vi "Run Command.vi"(2 "Line Index In":i32, 3 "Script":string) -> (0 "Line Index Out":i32, 1 "Done":bool)   [LabVIEW 2015]
doc: "Looks at a line and runs the appropriate command. Add new commands to this vi."
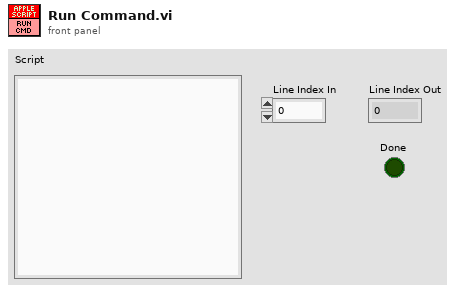
[diagram p1: front panel]
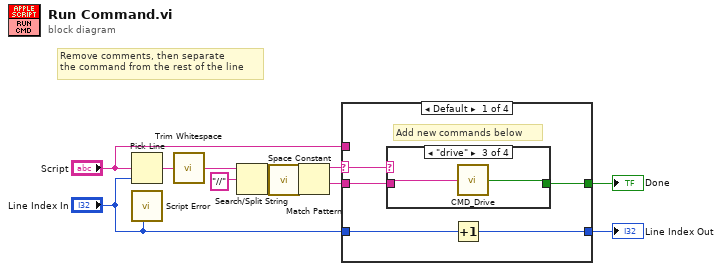
[diagram p0: block diagram]
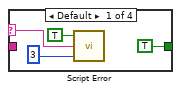
[diagram p2: hidden frame]
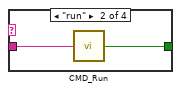
[diagram p3: hidden frame]
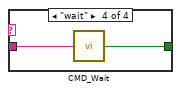
[diagram p4: hidden frame]
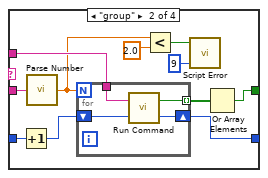
[diagram p5: hidden frame]
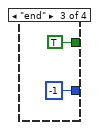
[diagram p6: hidden frame]
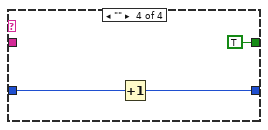
[diagram p7: hidden frame]
diagram:
  # "Remove comments, then separate\nthe command from the rest of the line"
  n1 = Pick Line(multi-line string="Script", line index="Line Index In") -> (output string=w6:string)  [unwired: 1 in]
  n2 = call "Script Error.vi"("Line Number"="Line Index In") -> ()  [unwired: 4 in, 1 out]
  n3 = call <vilib>:"Trim Whitespace.vi"("string"=w6) -> ("trimmed string"=w4:string)  [unwired: 1 in]
  n4 = Search/Split String(string=w4, search string/char (-)="//") -> (substring before match=w3:string)  [unwired: 1 in, 2 out]
  n5 = call <vilib>:"Space Constant.vi"() -> ("String"=w11:string)
  n6 = Match Pattern(string=w3, regular expression=w11) -> (before substring=w2:string, after substring=w1:string)  [unwired: 1 in, 2 out]
  n7 = case shown="Default" w2 {
    selector: w2 -> [w14 _ _ _]
    tunnel: "Script" -> [_ w37 _ _]
    tunnel: "Line Index In" -> [w16 w33 _ w45]
    tunnel: [w13 w35 TRUE ("Running") TRUE ("Running")] -> w9
    tunnel: [w15 w34 -1 ("Line Index Out") w44] -> w8
    tunnel: w1 -> [w12 w27 _ _]
    frame Default {
      # "Add new commands below"
      n8 = case shown="\"drive\"" w14 {
        selector: w14 -> [w17 _ _ _]
        tunnel: [TRUE w21 w23 w26] -> w13
        tunnel: w12 -> [_ w22 w24 w25]
        frame Default {
          n9 = call "Script Error.vi"("Error?"=TRUE, "Error Details"=w17, "Error Code"=3) -> ()  [unwired: 2 in, 1 out]
        }
        frame "run" {
          n10 = call "CMD_Run.vi"("Line"=w22) -> ("Done"=w21:bool)
        }
        frame "drive" {
          n11 = call "CMD_Drive.vi"("Line"=w24) -> ("Done"=w23:bool)
        }
        frame "wait" {
          n12 = call "CMD_Wait.vi"("Line"=w25) -> ("Done"=w26:bool)
        }
      }
      n13 = Increment(x=w16) -> (x+1=w15:i32)
    }
    frame "group" {
      n14 = Increment(x=w33) -> (x+1=w32:i32)
      n15 = call "Parse Number.vi"("String"=w27) -> ("Number"=w30:dbl)
      n16 = for {
        N: w30 -> [_]
        tunnel: w37 -> [w41]
        tunnel: [w40] -> w36 mode=indexing
        shift-right: [w39] -> w34
        shift-left: w32 -> [w38]
        n17 = call "Run Command.vi"("Line Index In"=w38, "Script"=w41) -> ("Line Index Out"=w39:i32, "Done"=w40:bool)
      }
      n18 = Less?(x=w30, y=2.0) -> (x < y?=w29:bool)
      n19 = call "Script Error.vi"("Error?"=w29, "Error Code"=9) -> ()  [unwired: 3 in, 1 out]
      n20 = Or Array Elements(Boolean array=w36) -> (logical OR=w35:bool)
    }
    frame "end" {
    }
    frame "" {
      n21 = Increment(x=w45) -> (x+1=w44:i32)
    }
  }
  "Line Index Out" <- w8
  "Done" <- w9
